vi "Make or Clean Directory.vi"(8 "Error In":errorcluster, 10 "Warn before delete? (T)":bool=TRUE, 11 "File Path to Make or Clean":path) -> (0 "Error Out":errorcluster, 3 "File Path out":path)   [LabVIEW 2014, in "i3-docs.lvlib"]
uses:
  i3-docs.lvlib
  <vilib>/Utility/error.llb/Error Cluster From Error Code.vi
  <vilib>/ErrorRing/Error Ring.xnode
panel:
  out "create tests":i32
  out "delete tests":i32
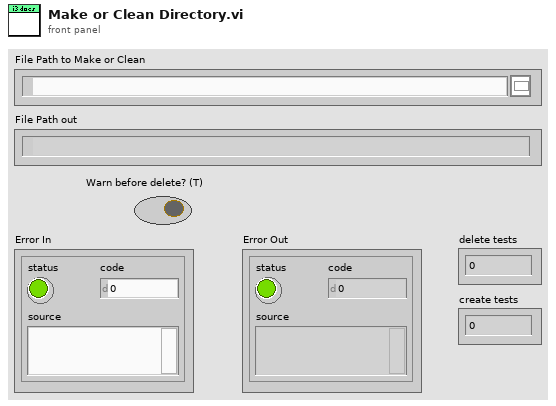
[diagram p1: front panel]
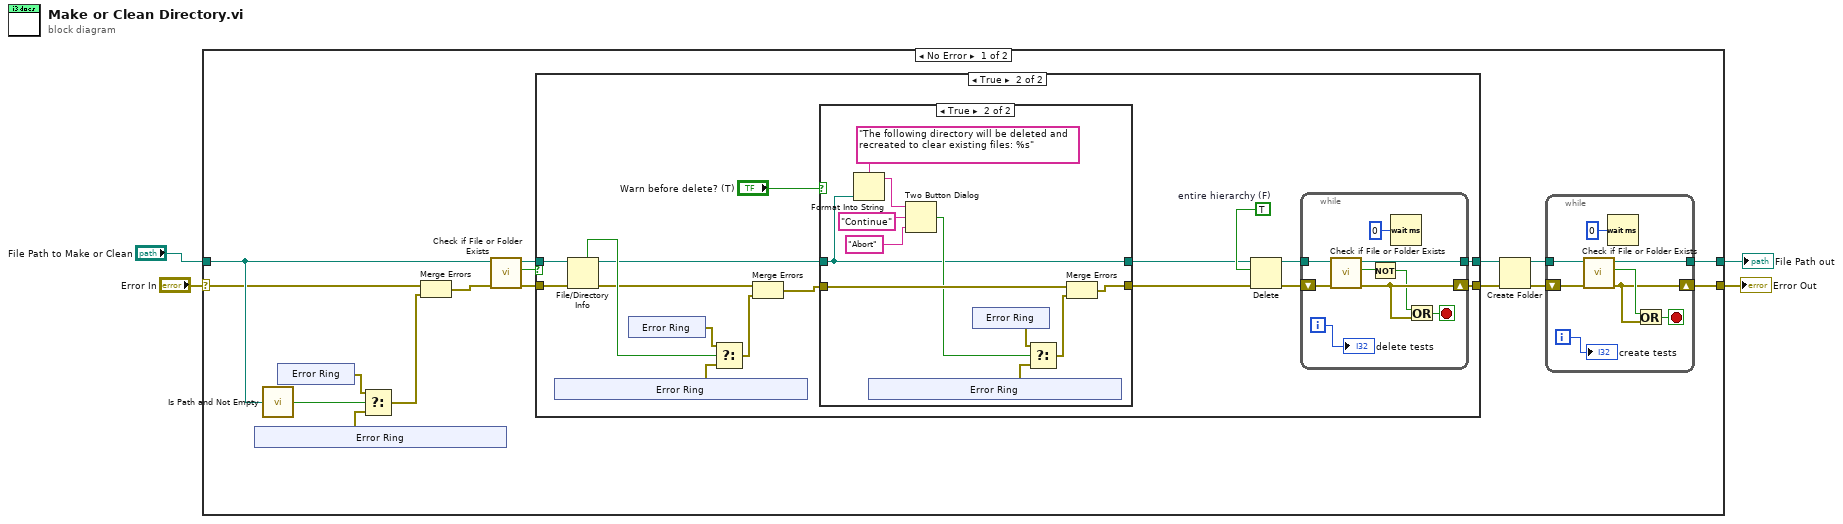
[diagram p0: block diagram]
diagram:
  n1 = case shown="No Error" "Error In" {
    selector: "Error In" -> [w11 w89]
    tunnel: "File Path to Make or Clean" -> [w15 w88]
    tunnel: [w7 w89] -> w3
    tunnel: [w5 w88] -> w1
    frame No Error {
      n2 = xnode "Error Ring"() -> ("error out"=w18:errorcluster)
      n3 = call <vilib>:"Is Path and Not Empty.vi"("path"=w15) -> ("Is Path and Not Empty?"=w20:bool)  [unwired: 4 in]
      n4 = xnode "Error Ring"() -> ("error out"=w19:errorcluster)
      n5 = Select(t=w19, s=w20, f=w18) -> (s? t:f=w17:errorcluster)
      n6 = Merge Errors(w11, w17) -> (w16:errorcluster)
      n7 = call <vilib>:"Check if File or Folder Exists.vi"("error in (no error)"=w16, "path"=w15) -> ("error out"=w12:errorcluster, "file or folder exists?"=w14:bool, "dup path"=w13:path)  [unwired: 7 in]
      n8 = case shown="True" w14 {
        tunnel: w13 -> [w29 w46]
        tunnel: w12 -> [w30 w47]
        tunnel: [w30 w37] -> w8
        tunnel: [w29 w36] -> w6
        frame False {
        }
        frame True {
          w40 = TRUE  # entire hierarchy (F)
          n9 = xnode "Error Ring"() -> ("error out"=w44:errorcluster)
          n10 = File/Directory Info(path=w46, error in=w47) -> (path out=w34:path, directory=w43:bool, error out=w41:errorcluster)  [unwired: 4 out]
          n11 = xnode "Error Ring"() -> ("error out"=w45:errorcluster)
          n12 = Select(t=w45, s=w43, f=w44) -> (s? t:f=w42:errorcluster)
          n13 = Merge Errors(w41, w42) -> (w33:errorcluster)
          n14 = case shown="True" "Warn before delete? (T)" {
            tunnel: [w49 w56] -> w35
            tunnel: w34 -> [w48 w50]
            tunnel: w33 -> [w49 w55]
            tunnel: [w48 w50] -> w31
            frame False {
            }
            frame True {
              n15 = Format Into String(format string="The following directory will be deleted and recreated to clear existing files: %s", w50) -> (resulting string=w54:string)  [unwired: 2 in, 1 out]
              n16 = xnode "Error Ring"() -> ("error out"=w59:errorcluster)
              n17 = Two Button Dialog(message=w54, 1:"Abort" ("F button name (\"Cancel\")"), 2:"Continue" ("T button name (\"OK\")")) -> (T button?=w53:bool)
              n18 = xnode "Error Ring"() -> ("error out"=w58:errorcluster)
              n19 = Select(t=w58, s=w53, f=w59) -> (s? t:f=w60:errorcluster)
              n20 = Merge Errors(w55, w60) -> (w56:errorcluster)
            }
          }
          n21 = Delete(path (use dialog)=w31, entire hierarchy (F)=w40, error in=w35) -> (deleted path=w38:path, error out=w39:errorcluster)  [unwired: 2 in, 1 out]
          n22 = while {
            shift-right: [w75] -> w37
            shift-left: w39 -> [w74]
            tunnel: w38 -> [w73]
            tunnel: [w72] -> w36
            i -> [w68]
            stop <- w70 stop-if-true
            n23 = call <vilib>:"Check if File or Folder Exists.vi"("error in (no error)"=w74, "path"=w73) -> ("error out"=w75:errorcluster, "file or folder exists?"=w71:bool, "dup path"=w72:path)  [unwired: 7 in]
            n24 = Not(x=w71) -> (.not. x?=w69:bool)
            n25 = Wait (ms)(milliseconds to wait=u32 0) -> ()  [unwired: 1 out]
            n26 = Or(x=w69, y=w75) -> (x .or. y?=w70:bool)
            "delete tests" <- w68
          }
        }
      }
      n27 = Create Folder(path (use dialog)=w6, error in=w8) -> (created path=w9:path, error out=w10:errorcluster)  [unwired: 1 in, 1 out]
      n28 = while {
        shift-right: [w23] -> w7
        shift-left: w10 -> [w28]
        tunnel: w9 -> [w27]
        tunnel: [w26] -> w5
        i -> [w22]
        stop <- w25 stop-if-true
        n29 = call <vilib>:"Check if File or Folder Exists.vi"("error in (no error)"=w28, "path"=w27) -> ("error out"=w23:errorcluster, "file or folder exists?"=w24:bool, "dup path"=w26:path)  [unwired: 7 in]
        n30 = Wait (ms)(milliseconds to wait=u32 0) -> ()  [unwired: 1 out]
        n31 = Or(x=w24, y=w23) -> (x .or. y?=w25:bool)
        "create tests" <- w22
      }
    }
    frame Error {
    }
  }
  "Error Out" <- w3
  "File Path out" <- w1
